vi "Save_On_Excel (SubVI).vi"(0 "NI_report in":refnum<class "NI_report.lvclass">, 1 "read buffer":string, 5 "report file path":path=path "C:/Users/Tulio/Documents/Testes/Backup excel/backup excel.xlsx", 7 "LED Measurement":dbl, 9 "Load Measurement":dbl, 11 "error in (no error)":errorcluster, 12 "Numeric":i32) -> (15 "error out":errorcluster)   [LabVIEW 2015]
uses:
  <vilib>/Utility/NIReport.llb/NI_report.lvclass
  <vilib>/addons/_office/NI_ReportGenerationToolkit.lvlib
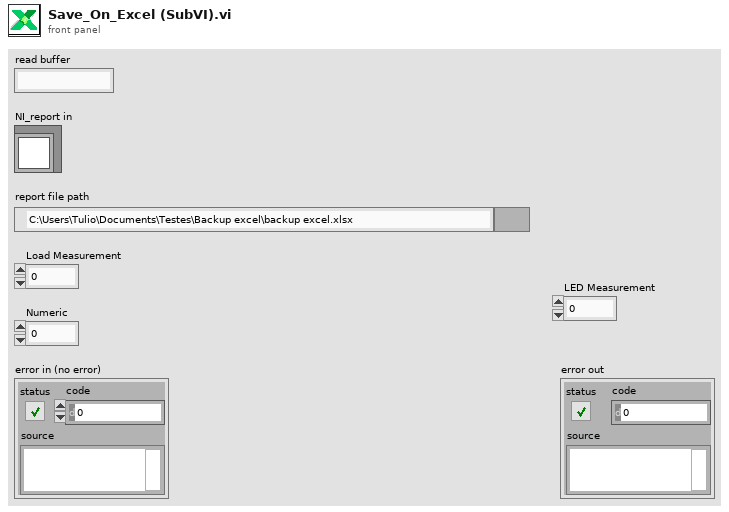
[diagram p1: front panel]
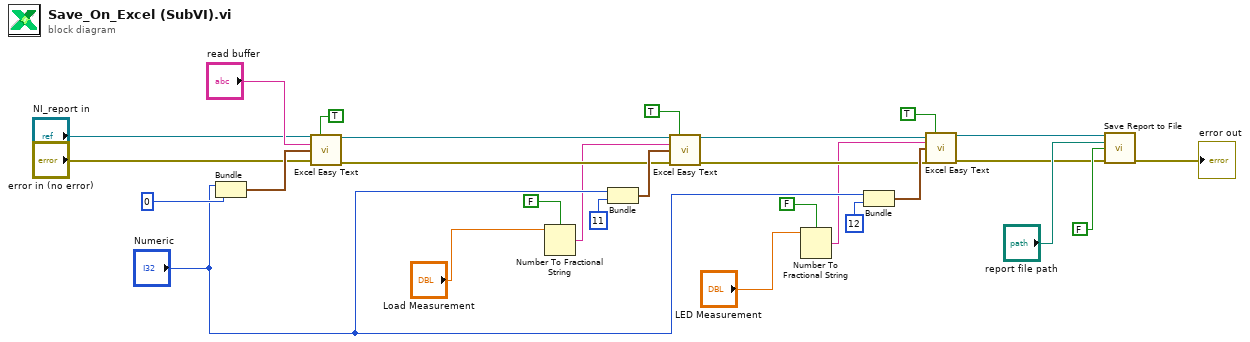
[diagram p0: block diagram]
diagram:
  n1 = Bundle("Numeric"="Numeric", "offset (0)"=0) -> (w16:cluster{"Numeric":i32, "offset (0)":i32})  [unwired: 1 in]
  n2 = call <vilib>:"Excel Easy Text.vi"("report in"="NI_report in", "border? (F)"=TRUE, "text"="read buffer", "start (-1, -1)"=w16, "error in (no error)"="error in (no error)") -> ("report out"=w19:refnum<class "NI_report.lvclass">, "error out"=w18:errorcluster)  [unwired: 6 in, 3 out]
  n3 = Number To Fractional String(use system decimal point (T)=FALSE, number="Load Measurement") -> (F-format string=w2:string)  [unwired: 2 in]
  n4 = Bundle("Numeric"="Numeric", "offset (0)"=11) -> (w21:cluster{"Numeric":i32, "offset (0)":i32})  [unwired: 1 in]
  n5 = call <vilib>:"Excel Easy Text.vi"("report in"=w19, "border? (F)"=TRUE, "text"=w2, "start (-1, -1)"=w21, "error in (no error)"=w18) -> ("report out"=w9:refnum<class "NI_report.lvclass">, "error out"=w8:errorcluster)  [unwired: 6 in, 3 out]
  n6 = Number To Fractional String(use system decimal point (T)=FALSE, number="LED Measurement") -> (F-format string=w3:string)  [unwired: 2 in]
  n7 = Bundle("Numeric"="Numeric", "offset (0)"=12) -> (w11:cluster{"Numeric":i32, "offset (0)":i32})  [unwired: 1 in]
  n8 = call <vilib>:"Excel Easy Text.vi"("report in"=w9, "border? (F)"=TRUE, "text"=w3, "start (-1, -1)"=w11, "error in (no error)"=w8) -> ("report out"=w6:refnum<class "NI_report.lvclass">, "error out"=w7:errorcluster)  [unwired: 6 in, 3 out]
  n9 = call-dynamic "Save Report to File.vi"("report in"=w6, "report file path"="report file path", "prompt to replace? (F)"=FALSE, "error in (no error)"=w7) -> ("error out"=→"error out":errorcluster)  [unwired: 10 in, 1 out]
